vi "Get Existing Traces.vi"(4 "Archive Database":path=path "\\\\localhost\\c__data", 6 "Logging Database":path=path "\\\\localhost\\c__data", 8 "error in (no error)":errorcluster, 11 "Shared Variable URLs":refnum<k21>[](array[refnum])) -> (0 "error out":errorcluster, 2 "Filtered Names":string[](array[string]), 3 "Filtered Shared Variable URLs":refnum<k21>[](array[refnum]))   [LabVIEW 2024]
doc: "Gets existing traces from the logging database and the archive database."
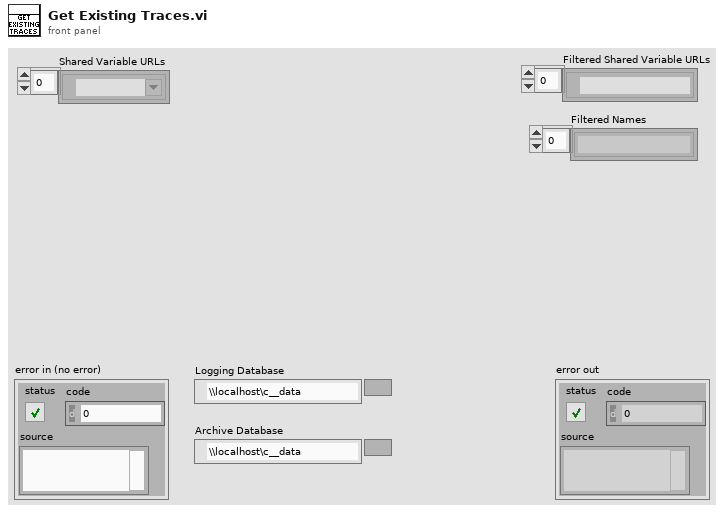
[diagram p1: front panel]
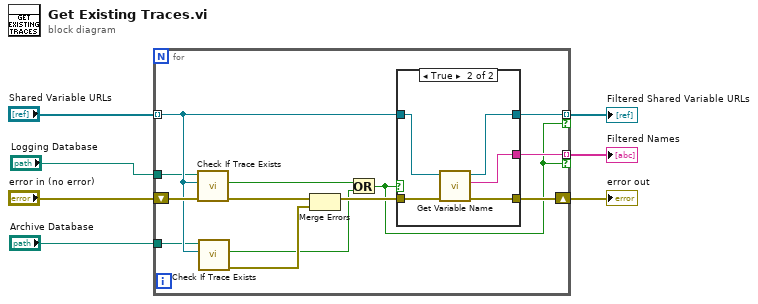
[diagram p0: block diagram]
diagram:
  n1 = for {
    shift-right: [w19] -> w6
    shift-left: "error in (no error)" -> [w18]
    tunnel: "Shared Variable URLs" -> [w17] mode=indexing
    tunnel: "Logging Database" -> [w12]
    tunnel: "Archive Database" -> [w11]
    tunnel: [w10] -> w2 mode=indexing if=w8
    tunnel: [w9] -> w1 mode=indexing if=w8
    n2 = call "Check If Trace Exists.vi"("error in (no error)"=w18, "Trace Name"=w17, "Database"=w12) -> ("error out"=w16:errorcluster, "Exist?"=w14:bool)  [unwired: 6 in, 1 out]
    n3 = call "Check If Trace Exists.vi"("Trace Name"=w17, "Database"=w11) -> ("error out"=w15:errorcluster, "Exist?"=w13:bool)  [unwired: 7 in, 1 out]
    n4 = Merge Errors(w16, w15) -> (w20:errorcluster)
    n5 = Or(x=w14, y=w13) -> (x .or. y?=w8:bool)
    n6 = case shown="True" w8 {
      tunnel: w17 -> [w21 w27]
      tunnel: w20 -> [w22 w26]
      tunnel: [w22 w25] -> w19
      tunnel: [w21 w24] -> w10
      tunnel: [_ w23] -> w9
      frame False {
      }
      frame True {
        n7 = call "Get Variable Name.vi"("error in (no error)"=w26, "Variable URL"=w27) -> ("error out"=w25:errorcluster, "Variable Name"=w23:string, "dup Variable URL"=w24:refnum<k21>)  [unwired: 7 in]
      }
    }
  }
  "error out" <- w6
  "Filtered Shared Variable URLs" <- w2
  "Filtered Names" <- w1
